vi "Release.vi"(8 "error in (no error)":errorcluster, 11 "QTab Class in":refnum<class "QTab Class.lvclass">) -> (0 "error out":errorcluster)   [LabVIEW 2020, in "QTab.lvlib" / "QTab Class.lvclass"]
uses:
  QTab Class.lvclass
  QTab Class.lvclass/QTab Class.ctl
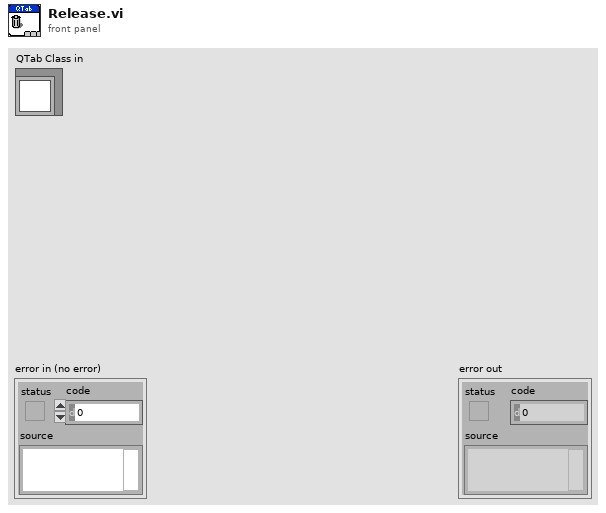
[diagram p1: front panel]
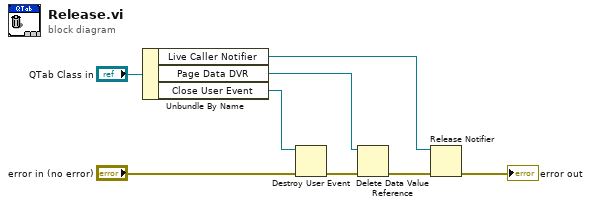
[diagram p0: block diagram]
diagram:
  n1 = Unbundle By Name("QTab Class in") -> ("Live Caller Notifier"=w7:refnum<notifier>, "Page Data DVR"=w4:refnum<data-value>, "Close User Event"=w2:refnum<user-event>)
  n2 = Destroy User Event(user event=w2, error in="error in (no error)") -> (error out=w3:errorcluster)
  n3 = Delete Data Value Reference(data value reference=w4, error in=w3) -> (error out=w5:errorcluster)  [unwired: 1 out]
  n4 = Release Notifier(notifier=w7, error in (no error)=w5) -> (error out=→"error out":errorcluster)  [unwired: 1 in, 2 out]
